vi "Get XBox.vi"(10 "Scalar":dbl=127.0, 11 "JoystickDevRefIn":T3) -> (1 "Buttons":T2, 2 "Axes":T1, 3 "JoystickDevRefOut":T3)   [LabVIEW 2013]
uses:
  <vilib>/Rock Robotics/WPI/Joystick/WPI_JoystickDevRef.ctl
  <vilib>/Rock Robotics/WPI/Joystick/WPI_JoystickDeviceEnum.ctl
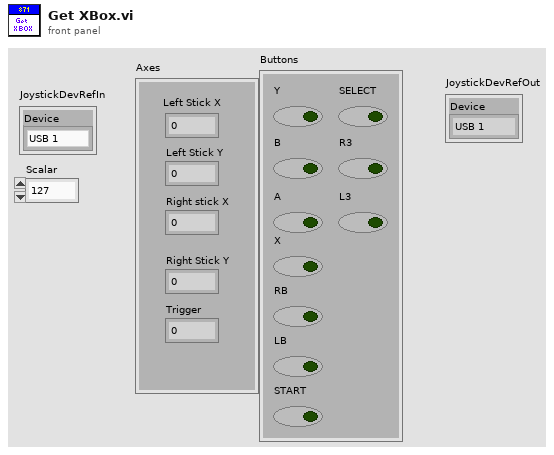
[diagram p1: front panel]
types:
  T1 = cluster{"Left Stick X":dbl, "Left Stick Y":dbl, "Right stick X":dbl, "Right Stick Y":dbl, "Trigger":dbl}
  T2 = cluster{"Y":bool, "B":bool, "A":bool, "X":bool, "RB":bool, "LB":bool, "START":bool, "SELECT":bool, "R3":bool, "L3":bool}
  T3 = typedef "WPI_JoystickDevRef.ctl" = cluster{"Device":T4}
  T4 = typedef "WPI_JoystickDeviceEnum.ctl" = enum16{"USB 1", "USB 2", "USB 3", "USB 4", "Kinect 1", "Kinect 2"}
  T5 = typedef "WPI_JoystickButtonState.ctl" = cluster{"Button 1":bool, "Button 2":bool, "Button 3":bool, "Button 4":bool, "Button 5":bool, "Button 6":bool, "Button 7":bool, "Button 8":bool, "Button 9":bool, "Button 10":bool, "Button 11":bool, "Button 12":bool}
  T6 = cluster{"axis 1 (x)":dbl, "axis 2 (y)":dbl, "axis 3 (throttle)":dbl, "axis 4":dbl, "axis 5":dbl, "axis 6":dbl}
  T7 = cluster{"axis 1 (x)":dbl, "axis 2 (y)":dbl, "axis 4":dbl, "axis 5":dbl, "axis 3 (throttle)":dbl}
  T8 = cluster{"Button 4":bool, "Button 2":bool, "Button 1":bool, "Button 3":bool, "Button 6":bool, "Button 5":bool, "Button 8":bool, "Button 7":bool, "Button 10":bool, "Button 9":bool}
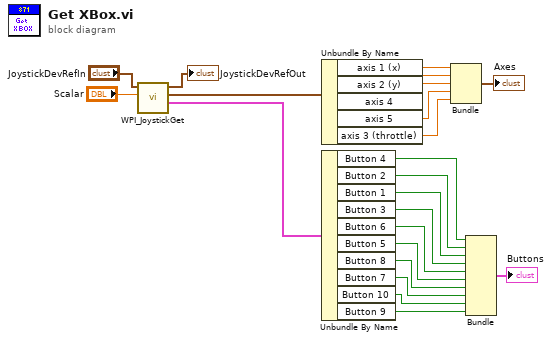
[diagram p0: block diagram]
diagram:
  n1 = call <vilib>:"WPI_JoystickGet.vi"("Scaler"="Scalar", "JoystickDevRef"="JoystickDevRefIn") -> ("Buttons"=w13:T5, "Axes"=w14:T6, "JoystickDevRef"=→"JoystickDevRefOut":T3)  [unwired: 3 in]
  n2 = Unbundle By Name(w14) -> ("axis 1 (x)"=w20:dbl, "axis 2 (y)"=w19:dbl, "axis 4"=w18:dbl, "axis 5"=w17:dbl, "axis 3 (throttle)"=w16:dbl)
  n3 = Unbundle By Name(w13) -> ("Button 4"=w12:bool, "Button 2"=w11:bool, "Button 1"=w10:bool, "Button 3"=w9:bool, "Button 6"=w8:bool, "Button 5"=w7:bool, "Button 8"=w6:bool, "Button 7"=w5:bool, "Button 10"=w4:bool, "Button 9"=w3:bool)
  n4 = Bundle("axis 1 (x)"=w20, "axis 2 (y)"=w19, "axis 4"=w18, "axis 5"=w17, "axis 3 (throttle)"=w16) -> (→"Axes":T7)  [unwired: 1 in]
  n5 = Bundle("Button 4"=w12, "Button 2"=w11, "Button 1"=w10, "Button 3"=w9, "Button 6"=w8, "Button 5"=w7, "Button 8"=w6, "Button 7"=w5, "Button 10"=w4, "Button 9"=w3) -> (→"Buttons":T8)  [unwired: 1 in]
